vi "parallel_loop-prob.vi"() -> ()   [LabVIEW 2019]
panel:
  out "Waveform Chart 2":dbl(graph)
  out "Waveform Chart":dbl(graph)
  in  "stop":bool
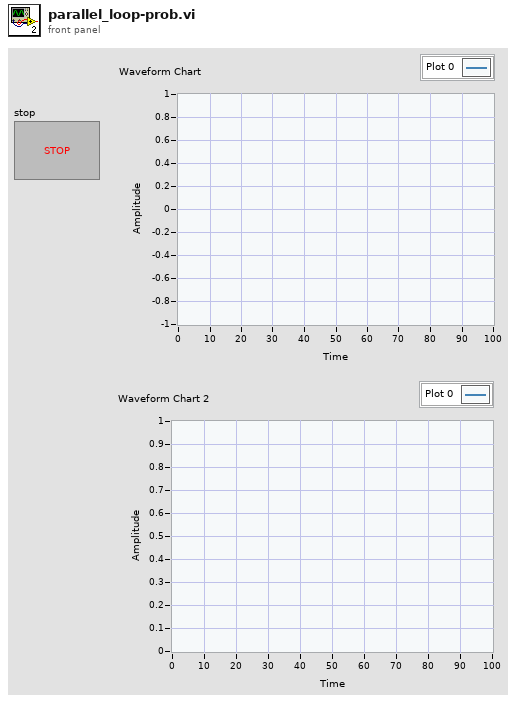
[diagram p1: front panel]
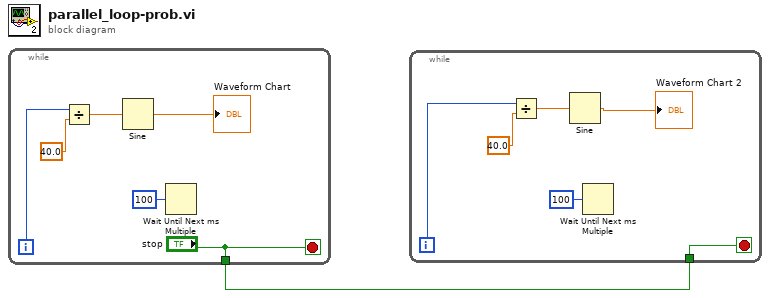
[diagram p0: block diagram]
diagram:
  n1 = while {
    tunnel: ["stop"] -> w1
    i -> [w5]
    stop <- "stop" stop-if-true
    n2 = Divide(x=w5, y=40.0) -> (x/y=w7:dbl)
    n3 = Sine(x=w7) -> (sin(x)=→"Waveform Chart":dbl)
    n4 = Wait Until Next ms Multiple(millisecond multiple=u32 100) -> ()  [unwired: 1 out]
  }
  n5 = while {
    tunnel: w1 -> [w8]
    i -> [w11]
    stop <- w8 stop-if-true
    n6 = Divide(x=w11, y=40.0) -> (x/y=w12:dbl)
    n7 = Sine(x=w12) -> (sin(x)=→"Waveform Chart 2":dbl)
    n8 = Wait Until Next ms Multiple(millisecond multiple=u32 100) -> ()  [unwired: 1 out]
  }
